vi "Enable Controls.vi"(8 "error in (no error)":errorcluster, 10 "Controls":bool, 11 "Simulated Entry Console in":refnum<class "Simulated Entry Console.lvclass">) -> (0 "error out":errorcluster, 3 "Simulated Entry Console out":refnum<class "Simulated Entry Console.lvclass">)   [LabVIEW 2012, in "Simulated Entry Console.lvlib" / "Simulated Entry Console.lvclass"]
uses:
  Simulated Entry Console.lvclass
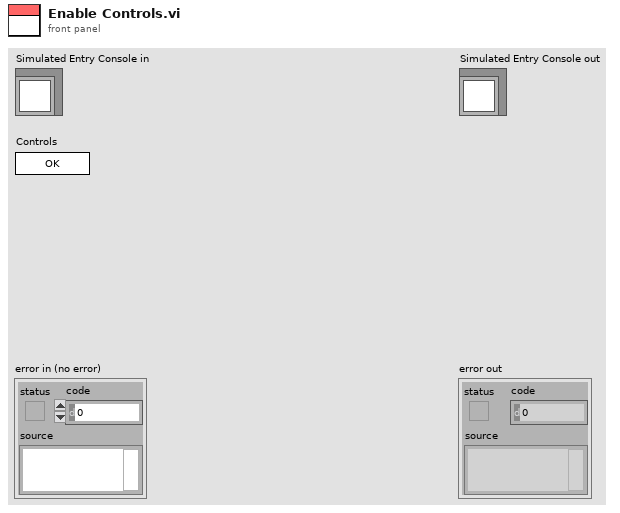
[diagram p1: front panel]
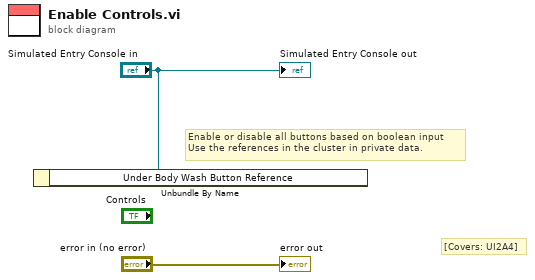
[diagram p0: block diagram]
diagram:
  # "Enable or disable all buttons based on boolean input\nUse the references in the cluster in private data."
  # "[Covers: UI2A4]"
  n1 = Unbundle By Name("Simulated Entry Console in") -> ()  [unwired: 1 out]
  "error out" <- "error in (no error)"
  "Simulated Entry Console out" <- "Simulated Entry Console in"
